vi "Data List.vi"(8 "error in (no error)":errorcluster, 9 "File Path":path, 10 "Table Infor":refnum<class "Data List.lvclass">[](array[class]), 11 "Data List Infor Interface in":refnum<class "Data List Infor Interface.lvclass">) -> (0 "error out":errorcluster, 3 "Data List Infor Interface out":refnum<class "Data List Infor Interface.lvclass">)   [LabVIEW 2020, in "Data List Infor Interface.lvclass"]
uses:
  Data List Infor Interface.lvclass
  Models/Data List/Data List.lvclass
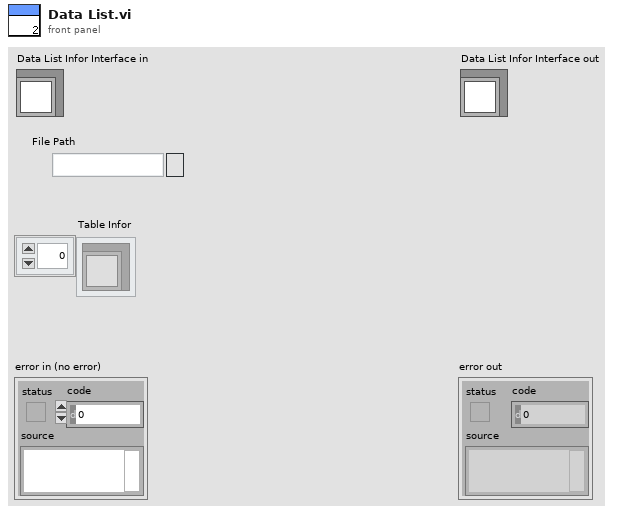
[diagram p1: front panel]
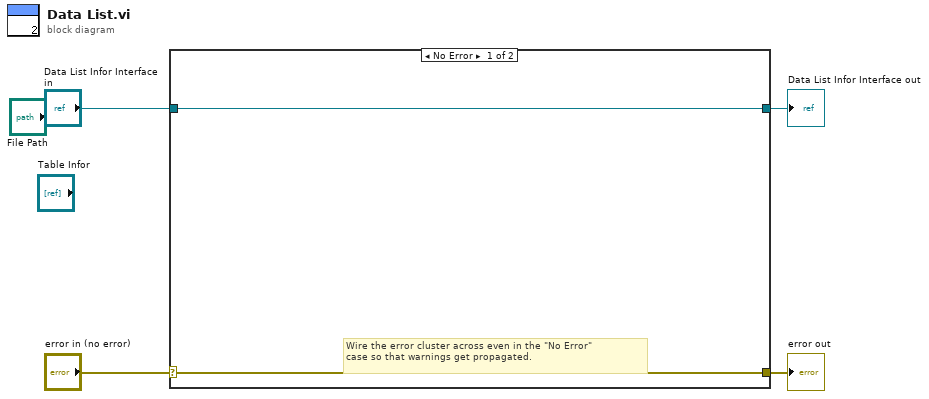
[diagram p0: block diagram]
diagram:
  n1 = case shown="No Error" "error in (no error)" {
    selector: "error in (no error)" -> [w5 w8]
    tunnel: [w5 w8] -> w3
    tunnel: [w6 w7] -> w1
    tunnel: "Data List Infor Interface in" -> [w6 w7]
    frame No Error {
      # "Wire the error cluster across even in the \"No Error\"\ncase so that warnings get propagated."
    }
    frame Error {
    }
  }
  "error out" <- w3
  "Data List Infor Interface out" <- w1
